vi "player movement data.vi"() -> ()   [LabVIEW 2013]
panel:
  out "ALL HY":string[](array[string])
  out "All DU":string[](array[string])
  out "All CJ opponents":string[](array[string])
  out "ALL CHEN JIN":string[](array[string])
  in  "top DU":string[](array[string])=["0 -1 0 -4 4 -4 1 -4 0\r\n", "1 -4 1 0 2 0 -3 0 2 0 -2 0 1 0 1 -4 4 -4 1 0 3 -2 0 -4 4 -4\r\n", "0 1 -4 4 -4 1\r\n", "0 3 0 -3 3 0 1 0 1 -4 4\r\n", "0 1 -4 0 1 -4\r\n", "0 3 -2 0 1 -4 1 0 2 0 4 0 4 0 -1 2 -1 0\r\n", "1 0 -1 0 2 0 4 -4\r\n", "-4\r\n", "-1 0 4\r\n", "0 1 -1 0 1 -4 0\r\n", "-1 0 1 -4 0 3 0 2 0 4 0 -4 4 -4 0 -1 0 -4 0 -2 0 4\r\n", "0 4 0\r\n", "0 4 -4 0 2 -1 0 2 0 4 -4 1 -4 4 0 3\r\n", "0 4 0 2 0\r\n", "1 0 -1 1 0 -4 1 -4 1 0 -4\r\n", "0 3 -2 0 -4\r\n", "2 -1 0 -4 4 -4 0 2 0 4\r\n", "1 0\r\n", "-1 0 -1 1 0 -4\r\n", "0 3 0\r\n", "0 -4 4 -4 0 -4 0 4 0 2 0 1 -4 4\r\n", "-1 0 1 -4\r\n", "-1 0 2 -1 0 2\r\n", "1 -1 0 4 -4 1\r\n", "-1 0 1 -4 4 -4 0 -4 4\r\n", "0 3 0 3 0 1 -1 0 1\r\n", "-1 0 4 0 4 -4 1 0 -4 0\r\n", "1 0 4\r\n", "0 -1 0 2 -1 0 -2 3 -2 0 -4 4 -4\r\n", "0 3 0\r\n", "2 -1 0 1 -4 4 -4 0 2 0\r\n", "0 4 -4 1 0 1 0 1 -4 0 2 0 4 0 4 -4 1\r\n", "1 -1 0 3 0 3 0 1 0 4\r\n", "0 -4 0 -2 0 -4\r\n", "0 -4 4 -4 0 -2 0 2 0\r\n", "-1 0 4 -4 0\r\n", "1 0 -1 2 0 4\r\n", "0 2 0 -2 0\r\n", "0 1 -4 0 -4 0 3 -2 0 -4 0 -4 4 -4 1\r\n"]
  in  "bottom CJ":string[](array[string])=["0 1 0 3 -2 3\r\n", "0 2 -2 3 -3 0 -3 3 -2 2 0 -4 4 -4 1 0 4 0 2 -2 0 4 0 4 0 2 -2 2\r\n", "0 -3 3 0 -2\r\n", "1 0 -2 0 4 0 1 0 -2 2 -2\r\n", "-2 0 3 0\r\n", "-4 0 -2 0 3 -3 0 -2 2 -2 0 -4 0 3 -2 0\r\n", "0 -3 4 0 1 0 -2\r\n", "-2\r\n", "-4 0\r\n", "-2 0 -3 4 -3 4 -4\r\n", "0 1 -4 0 -2 2 -2 0 -4 0 -3 3 -2 3 0 1 0\r\n", "0 3\r\n", "0 2 0 3 0 1 0 -2 2 -2 3 0\r\n", "-1 0 -1 1 0 4 -4 4 -4\r\n", "0 -3 4 -3 -2 2 -2 3 -2 2 -2 0\r\n", "2 0 -3 3\r\n", "0 3 0 -1 0\r\n", "0 3\r\n", "0 3 0 3\r\n", "-4 0 -4 1 -4\r\n", "2 -2 0 3 -3 0 1 0 -1 0 4 -3 0 2 -2 0\r\n", "0 1 0 4 -4 4 0\r\n", "0 1 0 -3 3 -3 0\r\n", "0 -3 4 0 -4 1 0 -2\r\n", "0 3 0 -2\r\n", "2 0 -3 3 -2 2 0 -2 0 -3 4 -3\r\n", "0 1 0 3 0\r\n", "0 3 0 -2\r\n", "-4 0 3 0 2 -1 0 3 0\r\n", "2 0 4 0 -2 2\r\n", "0 -3 4 -3 0 -2 2 -2 0 4\r\n", "0 3 -2 0 -3 4 0 3 0 1 -1 0 -1 0\r\n", "0 -3 4 -3 0\r\n", "2 0 3 -3 0 -4 0 -2\r\n", "-1 0 3 -3 0 1 0 4\r\n", "0 1 0\r\n", "0 -1 0 -1 1 -1 0\r\n", "0 -3 3 -3 0 1 -4 0 -1 0\r\n", "2 0 3 -2 0 -2 3 -2 0\r\n"]
  in  "top CJ":string[](array[string])=["0 3 0 1 0 -3 0 -3 3 0\r\n", "1 -4\r\n", "2 0 2 0 -1 0 -3\r\n", "0 4\r\n", "0 -1 2 -1 0 2 0 3 0 1 -4 1 0 -4 4 -4\r\n", "0 -1 0 -4 0 -2 0\r\n", "1 -1 1 0 -4\r\n", "-1 0 -4 0 1 0\r\n", "0 3\r\n", "-1 1 0 -4 1 0 -4 0 -1 2 0\r\n", "1 0 -1 0 2\r\n", "0 -1 -4 1 0 -3 3\r\n", "2 -1 0\r\n", "0 4 0 2 0 -3 0 1 -1 0 1 -4 4 -4 4 -4 0 3\r\n", "0 -4 4 -4 0 -1 2 0 3 -3 0 -3 3 0 -4 1 0 -3 0 3 -2\r\n", "0 3 0\r\n", "0 4 0 1 0 -4 4\r\n", "0 -1 0 4 0\r\n", "1 -1 0 4 0 2 -2 0 -4 1 -4 4 -3 0 -4 0 -3 3 0 -4 1 -1 2 -1 0 4\r\n", "0 3 0 4 -4 4 -4 1 -4 1 -4 4 -4 1 -4 0 -3 3\r\n", "", "0\r\n", "0 4 -4 0 -4 0 4 -4 0\r\n", "1 -4\r\n", "0 4\r\n", "0 1 -4 1 -4 0 -4 4 -4 0\r\n", "-2 2 0 -3 3 -3 0 3 0\r\n", "1 0 4 0\r\n", "0 3 0 1 0\r\n", "0 4 -4 0 -4 1 -4 0\r\n", "0\r\n", "0 -4 4 -4 0 -3 3 -2 0 2\r\n", "0 3 0 1 0 -4 4 0 -3 3 0 -4 0\r\n"]
  in  "bottom DU":string[](array[string])=["-2 0 3 0 -3 0 4 -4 0\r\n", "0 3\r\n", "0 4 -3 0 -4 1 0 4 -3 0\r\n", "0\r\n", "-2 0 3 -3 0 -4 1 -4 0 3 -3 4 -3 0 2 0 3\r\n", "0 3 0 1\r\n", "0 1 0 3\r\n", "0 3 -2 0 4\r\n", "0\r\n", "0 -3 4 0 2 -2 0 -3 0 3 -2 3 -3 4\r\n", "0 -3 4 -3 0\r\n", "-2 0 -2 2 0\r\n", "0 3 -2\r\n", "0 4 -3 0 3 -2 0 -3 4 -3 0 3 -2 2 -2 0 4 0\r\n", "2 0 1 -4 0 3 0 -4 4 0 -4 4 0 2 0 4 0 -3 4 -3 0 -4 0 4\r\n", "0 4\r\n", "-2 0 -2 0 3 0\r\n", "0 3 0 -2 3\r\n", "0 4 0 4 -4 0 2 0 -4 4 -3 0 -2 2 -2 0 4 -3 0 2 0 3 0\r\n", "0 4 -3 0 1 -1 0 3 0 -2 2 -2 0 -3 4 -3 0 4 -4 1 0\r\n", "", "0 -3\r\n", "2 0 3 0 1 0 -2 3\r\n", "0\r\n", "1 -1 0\r\n", "0 -2 3 0\r\n", "0 1 0 4 0 4 -4 4\r\n", "0 1 -1 0 3\r\n", "0 2 -2 3 -3 4\r\n", "-2 2 0 -2 3\r\n", "0 -1\r\n", "0 4 -4 4 0 3 0 -2 0 -4 0 1 -4\r\n", "-2 0 4 0 -3 3 0 -2 2 -2 0 -4 0 4 0\r\n"]
  in  "top CJ":string[](array[string])=["0 1 -1 1 -1 1 0\r\n", "1 0\r\n", "2 -2 0 3 0 4 0 -1 0 -1\r\n", "0 4 -4 1\r\n", "0 4 -4 0 4 0 -4 1 -1 0 -3 3 0 4 -4 0 -1 0 4\r\n", "-4 0 -3 0 -4 0 2 0 4 0 -2 0 -1 1 0 4 -4\r\n", "0 -1 1 0\r\n", "0 4 0 1 -1 0\r\n", "0 2 -1 0 -4 4 -4 0 -1 1\r\n", "2 0 2 0 2 0 -3 0 4 -4 1 0\r\n", "1 0 4 0 2 0 -2 3 -2 0 4 -4 0\r\n", "0 4 0 2 0 4\r\n", "-1 1 -1 2\r\n", "0 4 -4 0 -1 2 0 -4 1 -4 4 -4 0 -4 4 -3 0 4 -4 1 0 3\r\n", "0 -1\r\n", "2 0 2 0 2\r\n", "0 3 -2 0 -1 1 -1 0 -3 0\r\n", "2 0\r\n", "0 3\r\n", "0 4 -4 1 0 3 -2 2 -2 2 0 4 0 4 0\r\n", "-4 0 -2 0 2 0 4 -4 1 -4 1 0 1\r\n", "0\r\n", "0\r\n", "0 4\r\n", "-2 2 0 -1 0 4 -4 1 0 1 -1 0 1 0 4 0 -4 4 0 2 0\r\n", "0 -1\r\n", "1 0 4 0 -2 0 -2 0 1\r\n", "2 0 -4 0 4 -3 0 1\r\n", "0 -1 1 0 -4 0\r\n", "-4 1 0 -4 0 -1 1\r\n", "0 4 0 2\r\n", "0 3 2 3\r\n", "2 0 -4 1 -4 4 -3 0 2 -1 1 -1 0 4 0 -3 0 2 0 3 -2 2 0 3\r\n", "0 1\r\n"]
  in  "bottom HY":string[](array[string])=["-2 2 -2 0 -1\r\n", "0 4 -3 0\r\n", "0 1 0 -1 1\r\n", "-4 0\r\n", "-2 0 3 0 1 0 3 -2 0 -1 0 4 0 3 0 -3 3 -3\r\n", "0 4 0 -2 0 1 0 -4 4 -3 0 1 0 4 0 -4 1 0 3 -3 0\r\n", "0 -1 2\r\n", "2 0 -3 4 0\r\n", "-4 0 -3 3 -3 0 -3 3 0 -2 3 0\r\n", "0 -1 1 -4 4 -3 0 3 0\r\n", "0 -1 2 0 3 0 1 -4 4 0 2 0\r\n", "2 -2 0 -4 0 -4 4 0 -4\r\n", "1 -1 2 -1\r\n", "2 0 -2 0 4 0 2 0 3 0 -2 0 -4\r\n", "1 -1 0 -1\r\n", "0 1 -4 1\r\n", "0 4 0 -1 1 -1 0\r\n", "0 3\r\n", "-2 0\r\n", "1 -4 0 -2 0 4 0 -4 0 4 -3 0 1 -4 0 1\r\n", "0 -3 3 -2 0 3 0 -2 2\r\n", "1 0\r\n", "2\r\n", "0 -4\r\n", "0 4 0 -4 0 -3 3 -3 0 -2 0 -2 0 4 0 -1 1 0 3 0 -4 1 -4 0 4\r\n", "2 0 -1 1\r\n", "0 2 0 4 0 4 -4 0 -1 2\r\n", "0 3 -2 0 3 -2\r\n", "1 0 -3 3 0 -4\r\n", "0 -3 3 0 -1 0\r\n", "2 -2 0 1\r\n", "-4 1 -4 1 -4 0\r\n", "0 4 0 2 0 -4 1 2 -1 0 4 0 1 0 4 -4 4 0 -4 4 0\r\n", "-2 0 3 0 -2 0\r\n"]
  in  "top HY":string[](array[string])=["0 4 0 4 0 4 0 4 0 -2 3 0 3 0 4 0\r\n", "-4 -1\r\n", "-2 0 1 0 -4 4\r\n", "0 4\r\n", "-2 2 0 -1 -4 1 0 3 0\r\n", "-1 0 -1 2\r\n", "0 -1 1 0 4 0 3 -2 0 -2 3 -2 0 4 0 -2 2\r\n", "2 -1 0 4\r\n", "0 4 0 2 0 -2 0\r\n", "1 -1 0 3 0 -4 4 -4 0\r\n", "2 -1 0 3 -2 0 -3 0 3 0 -3 0\r\n", "0 4 0 4 -4 1 -1 0 -3 0 1 -4 1 0 4 0 -4 0 -4 4 -4 1\r\n", "0 -4 1 0 -4 4\r\n", "0 4 0 -2 2 -2 2 -2 2\r\n", "-2 2 -1 0 4 0 2 0 4 0 2 -2 0 4\r\n", "1 0 -1 0 -1 0 1 -1\r\n", "-2 2 -2 3\r\n", "1 0 -1 0 -1 2 0 2 -2 0 -4 0\r\n", "-2 2 0 3 -2 2\r\n", "0\r\n", "1 -1 0 3\r\n", "0 4 0\r\n", "-2 0 1 -4 0 -3 0\r\n", "1 0 -1 2 -1 1 -4\r\n", "0 4\r\n", "-2 0 -1 1\r\n", "0 3 0 3 0 3 -2\r\n", "-4 0 -4 4\r\n", "0 4 0 -4 0 -4\r\n", "-2 2 0 4 -4 0 2 -2\r\n"]
  in  "bottom CJ":string[](array[string])=["2 0 3 -3 0 3 -3 0 4 0 4 0 -2 0 3\r\n", "0 -1\r\n", "0 4 0 3 0\r\n", "-4 0\r\n", "0 3 0 2 0\r\n", "0 1\r\n", "-2 0 -3 3 -2 0 3 -3 0 -4 4 0 1 0 -2 3 0 -3 4 0 1\r\n", "0 -1 2 0\r\n", "-4 0 4 -4 0 -2\r\n", "0 -1 0 4 -3 0 2 -2 3\r\n", "0 3 0 1 0 3 -3 0 1 0 1\r\n", "2 0 3 0 2 0 -3 4 0 -3 4 0 2 0 3 0 2\r\n", "0 3 0\r\n", "-4 0 2\r\n", "0 1 0 1 -4 4 -3 0 3 -3 4 0 2 -2\r\n", "0 4 0 2 -2 0\r\n", "0 4 0\r\n", "0 1 -4 4 -4 0 -3 3 0 -2 3\r\n", "0 1 -4 0 -4\r\n", "0 2 0 4\r\n", "0 -1 0 4\r\n", "-4 0 -2 3\r\n", "0 3 0 1 -4 0 -4\r\n", "0 1 -1 2\r\n", "0 3 -3 0\r\n", "0 4 0 -1 2\r\n", "-4 0 -4 4 0 4 0 -4 4\r\n", "0 3 -2 0\r\n", "0 3 -2 3 -2 2\r\n", "0 1 0 4\r\n"]
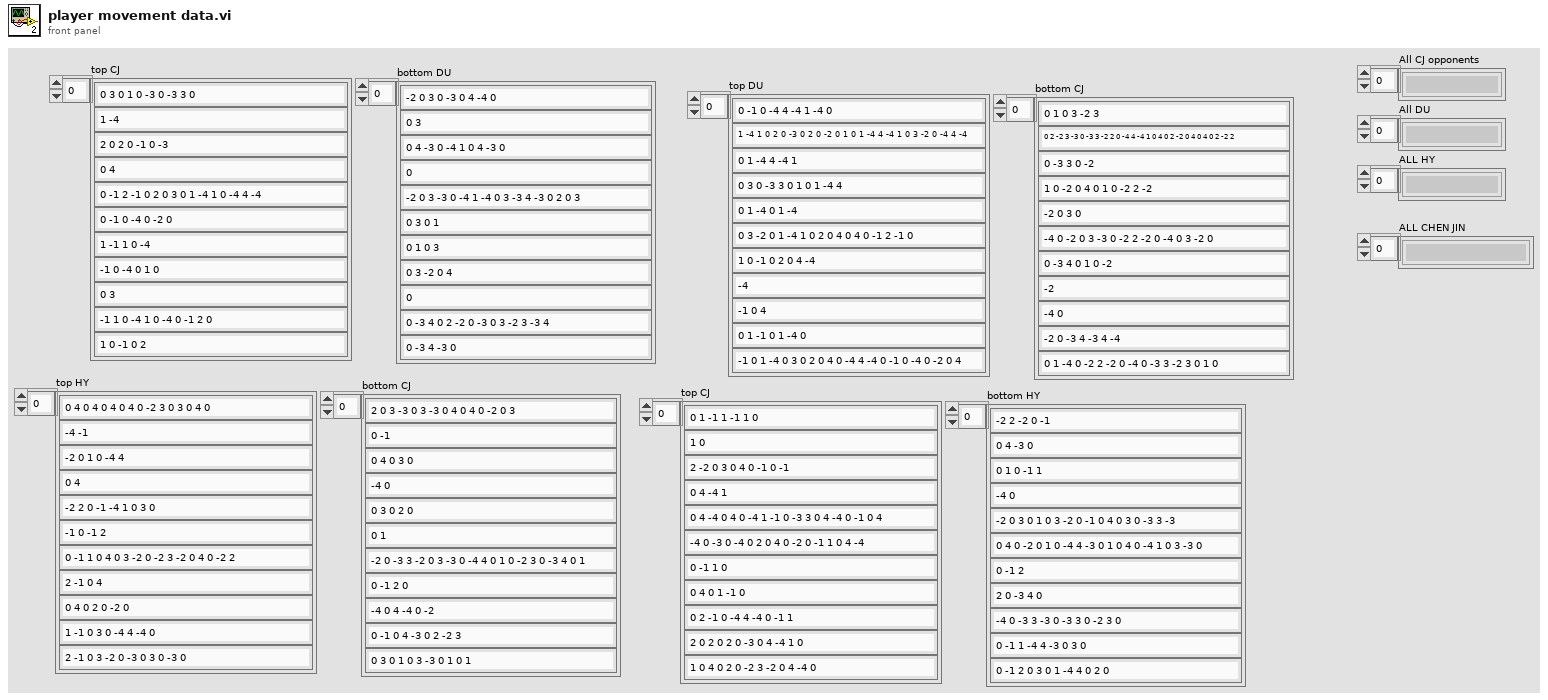
[diagram p1: front panel]
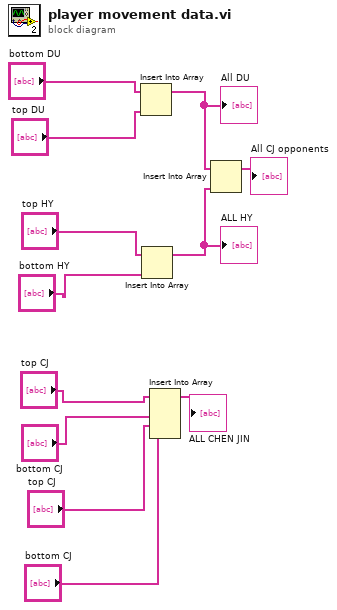
[diagram p0: block diagram]
diagram:
  n1 = Insert Into Array(array="bottom DU", new element="top DU") -> (w3:string[])  [unwired: 1 in]
  "All DU" <- w3
  n2 = Insert Into Array(array="top HY", new element="bottom HY") -> (w2:string[])  [unwired: 1 in]
  "ALL HY" <- w2
  n3 = Insert Into Array(array="top CJ", new element #1="bottom CJ", new element #2="top CJ", new element #3="bottom CJ") -> (→"ALL CHEN JIN":string[])  [unwired: 1 in]
  n4 = Insert Into Array(array=w3, new element=w2) -> (→"All CJ opponents":string[])  [unwired: 1 in]
